vi "fgv_ref-btn.vi"(7 "cmd":T2, 11 "ref":T1) -> (3 "ref 2":T1)   [LabVIEW 2019]
uses:
  _ctrl/rw.ctl
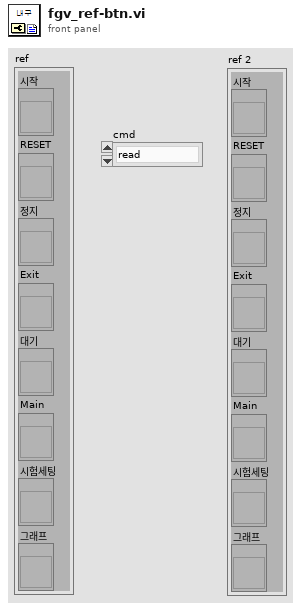
[diagram p1: front panel]
types:
  T1 = cluster{"시작":refnum<vi>, "RESET":refnum<vi>, "정지":refnum<vi>, "Exit":refnum<vi>, "대기":refnum<vi>, "Main":refnum<vi>, "시험세팅":refnum<vi>, "그래프":refnum<vi>}
  T2 = typedef "rw.ctl" = enum16{"read", "write"}
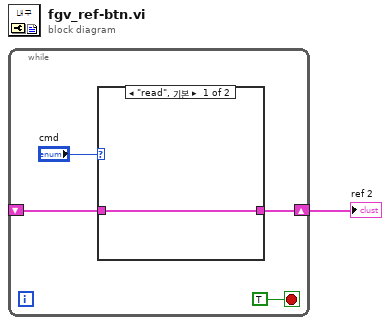
[diagram p0: block diagram]
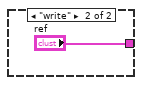
[diagram p2: hidden frame]
diagram:
  n1 = while {
    shift-right: [w3] -> w1
    shift-left: _ -> [w2]
    stop <- TRUE stop-if-true
    n2 = case shown="\"read\", 기본" "cmd" {
      tunnel: [w6 "ref"] -> w3
      tunnel: w2 -> [w6 _]
      frame "read", Default {
      }
      frame "write" {
      }
    }
  }
  "ref 2" <- w1
